vi "ELVIS III v1.0 Write AO Block Bank B DMA.vi"(8 "error in (no error)":errorcluster, 9 "AO FIFO Clock Divisor":u32, 10 "Bank Data":T1 caption="DO (N Samples) Configuration", 11 "FPGA Reference out":T3) -> (0 "error out":errorcluster)   [LabVIEW 2021]
uses:
  <vilib>/myRIO/Common/Instrument Driver Framework/Utilities/typedefs/Generic FPGA Reference.ctl
  <vilib>/myRIO/Common/Instrument Driver Framework/ELVIS III v1.0/AO Block/typedefs/ELVIS III AO Block Bank Data.ctl
  <vilib>/myRIO/Common/Instrument Driver Framework/ELVIS III v1.0/AO Block/typedefs/ELVIS III AO Block Channels FPGA Reference.ctl
  <vilib>/Utility/error.llb/Error Cluster From Error Code.vi
  <vilib>/rvi/errors/niLvFpgaAdjustHostInterfaceError.vi
  <vilib>/rvi/interface/nirviReadWriteControl/nirviReadWriteControl.xnode
  <vilib>/rvi/interface/nirviMethod/nirviMethod.xnode
  <vilib>/rvi/interface/Simulation/niFpgaSimulationCallBeginRW.vi
  <vilib>/FPGAPlugInAG/Dynamic/niLvFpga_WriteFifo_Dynamic.vi
  <vilib>/rvi/errors/niLvFpgaMergeErrorWithErrorCode.vi
  NiFpgaLv.dll
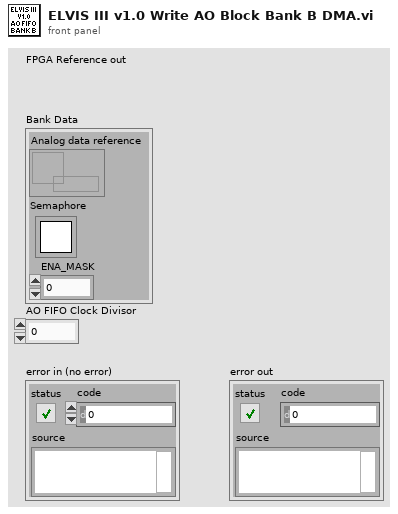
[diagram p1: front panel]
types:
  T1 = typedef "ELVIS III AO Block Bank Data.ctl" = cluster{"Analog data reference":refnum<data-value>, "Semaphore":T2, "ENA_MASK":u8}
  T2 = typedef "Semaphore RefNum" = refnum<k1>
  T3 = typedef "Generic FPGA Reference.ctl" = refnum<k20>
  T4 = typedef "ELVIS III AO Block Channels FPGA Reference.ctl" = refnum<k20>
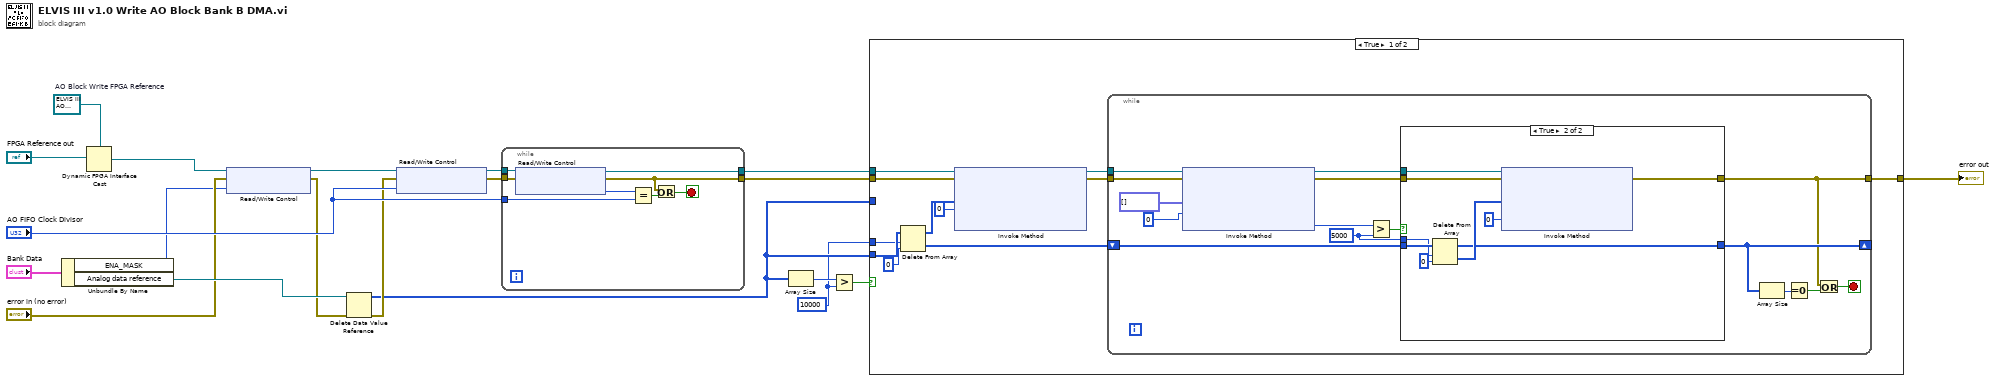
[diagram p0: block diagram]
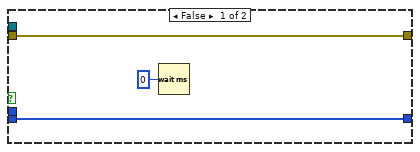
[diagram p2: hidden frame]
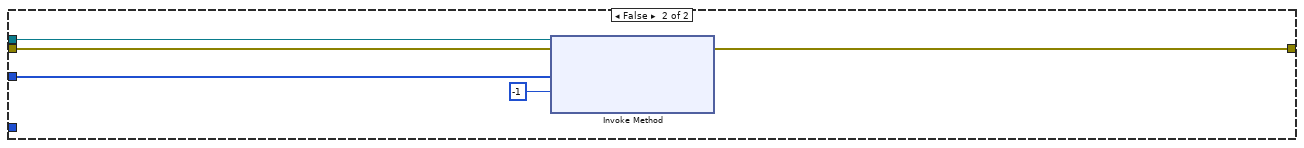
[diagram p3: hidden frame]
diagram:
  w7 = 10000 ("y")
  w16 = T4 refnum  # AO Block Write FPGA Reference
  n1 = Unbundle By Name("Bank Data") -> ("ENA_MASK"=w1:u8, "Analog data reference"=w13:refnum<data-value>)
  n2 = Dynamic FPGA Interface Cast(Session In=w16, Type="FPGA Reference out") -> (Session Out=w6:T4)
  n3 = xnode "Read/Write Control"("FPGA VI Reference In"=w6, "error in"="error in (no error)", "AO.B.DMA_ENA"=w1) -> ("FPGA VI Reference Out"=w5:T4, "error out"=w3:errorcluster)
  n4 = Delete Data Value Reference(data value reference=w13, error in=w3) -> (data value=w9:i32[], error out=w11:errorcluster)
  n5 = xnode "Read/Write Control"("FPGA VI Reference In"=w5, "error in"=w11, "AO.B.DMA_CNTR"="AO FIFO Clock Divisor") -> ("FPGA VI Reference Out"=w20:T4, "error out"=w19:errorcluster)
  n6 = while {
    tunnel: w20 -> [w28]
    tunnel: [w27] -> w18
    tunnel: [w23] -> w17
    tunnel: w19 -> [w26]
    tunnel: "AO FIFO Clock Divisor" -> [w24]
    stop <- w21 stop-if-true
    n7 = xnode "Read/Write Control"("FPGA VI Reference In"=w28, "error in"=w26) -> ("FPGA VI Reference Out"=w27:T4, "error out"=w23:errorcluster, "AO.B.DMA_CNTR"=w25:u32)
    n8 = Equal?(x=w25, y=w24) -> (x = y?=w22:bool)
    n9 = Or(x=w23, y=w22) -> (x .or. y?=w21:bool)
  }
  n10 = Array Size(array=w9) -> (size(s)=w8:i32)
  n11 = Greater?(x=w8, y=w7) -> (0:w10:bool)
  n12 = case shown="True" w10 {
    tunnel: w18 -> [w36 w70]
    tunnel: w17 -> [w38 w69]
    tunnel: w9 -> [_ w67]
    tunnel: [w30 w66] -> w2
    tunnel: w9 -> [w34 _]
    tunnel: w7 -> [w33 _]
    frame True {
      n13 = Delete From Array(array=w34, length=w33, index=0) -> (deleted portion=w31:i32[], array with subset deleted=w32:i32[])
      n14 = xnode "Invoke Method"("FPGA VI Reference In"=w36, "Data"=w32, "Timeout (ms)"=0) -> ("FPGA VI Reference Out"=w35:T4)  [unwired: 1 in, 2 out]
      n15 = while {
        shift-right: [w44] -> _
        shift-left: w31 -> [w53]
        tunnel: w38 -> [w52]
        tunnel: w35 -> [w51]
        tunnel: [w41] -> w30
        stop <- w39 stop-if-true
        w46 = u32 5000 ("y")
        n16 = xnode "Invoke Method"("FPGA VI Reference In"=w51, "error in"=w52, "Data"=fxp<+/-,20,5>[] [] ("Array"), "Timeout (ms)"=0) -> ("FPGA VI Reference Out"=w42:T4, "error out"=w43:errorcluster, "Empty Elements Remaining"=w48:u32)
        n17 = Greater?(x=w48, y=w46) -> (0:w47:bool)
        n18 = case shown="True" w47 {
          tunnel: w53 -> [w56 w64]
          tunnel: [w56 w60] -> w44
          tunnel: w46 -> [_ w63]
          tunnel: [w54 w62] -> w41
          tunnel: w43 -> [w54 w58]
          tunnel: w42 -> [_ w57]
          frame False {
            n19 = Wait (ms)(milliseconds to wait=u32 0) -> ()  [unwired: 1 out]
          }
          frame True {
            n20 = Delete From Array(array=w64, length=w63, index=0) -> (deleted portion=w61:i32[], array with subset deleted=w60:i32[])
            n21 = xnode "Invoke Method"("FPGA VI Reference In"=w57, "error in"=w58, "Data"=w61, "Timeout (ms)"=0) -> ("error out"=w62:errorcluster)  [unwired: 2 out]
          }
        }
        n22 = Array Size(array=w44) -> (size(s)=w45:i32)
        n23 = Equal To 0?(x=w45) -> (x = 0?=w40:bool)
        n24 = Or(x=w41, y=w40) -> (x .or. y?=w39:bool)
      }
    }
    frame False {
      n25 = xnode "Invoke Method"("FPGA VI Reference In"=w70, "error in"=w69, "Data"=w67, "Timeout (ms)"=-1) -> ("error out"=w66:errorcluster)  [unwired: 2 out]
    }
  }
  "error out" <- w2
